vi "Digital Output Control VI.vi"(11 "Car Wash Indicators":T1) -> ()   [LabVIEW 2021]
doc: "This VI receives the boolean cluster of the front panel indicators and converts the data to show the same indicators in the BNC-2120 digital outputs LEDs."
uses:
  Controls/Car Wash Indicators.ctl
  <vilib>/DAQmx/write.llb/DAQmx Write (Digital 1D U32 NChan 1Samp).vi
  <vilib>/DAQmx/create/channels.llb/DAQmx Create Channel (DO-Digital Output).vi
  <vilib>/DAQmx/miscellaneous.llb/DAQmx Fill In Error Info.vi
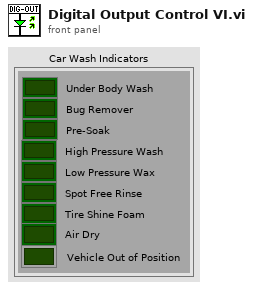
[diagram p1: front panel]
types:
  T1 = typedef "Car Wash Indicators.ctl" = cluster{"Vehicle Out of Position":bool, "Under Body Wash":bool, "Bug Remover":bool, "Pre-Soak":bool, "High Pressure Wash":bool, "Low Pressure Wax":bool, "Spot Free Rinse":bool, "Tire Shine Foam":bool, "Air Dry":bool}
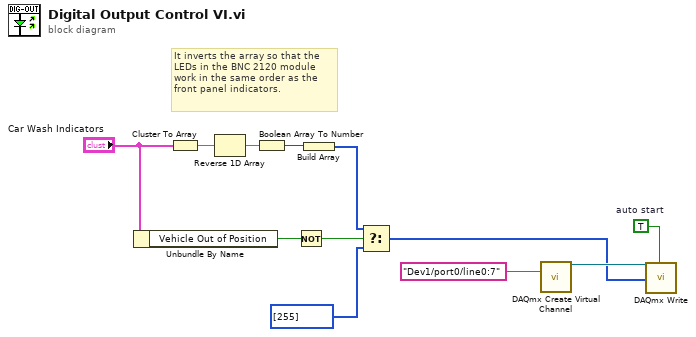
[diagram p0: block diagram]
diagram:
  w10 = TRUE  # auto start
  # "It inverts the array so that the LEDs in the BNC 2120 module work in the same order as the front panel indicators."
  n1 = Unbundle By Name("Car Wash Indicators") -> ("Vehicle Out of Position"=w5:bool)
  n2 = Cluster To Array(cluster="Car Wash Indicators") -> (array=w8:bool[])
  n3 = Reverse 1D Array(array=w8) -> (reversed array=w7:bool[])
  n4 = Boolean Array To Number(Boolean array=w7) -> (number=w11:u32)
  n5 = Not(x=w5) -> (.not. x?=w4:bool)
  n6 = Build Array(w11) -> (w3:u32[])
  n7 = Select(t=w3, s=w4, f=u32[] [255]) -> (s? t:f=w2:u32[])
  n8 = call-poly <vilib>:"DAQmx Create Virtual Channel.vi"("lines"="Dev1/port0/line0:7") -> ("task out"=w9:refnum<k21>)  [unwired: 13 in, 1 out]
  n9 = call-poly <vilib>:"DAQmx Write.vi"("task/channels in"=w9, "auto start"=w10, "data"=w2) -> ()  [unwired: 10 in, 3 out]
